vi "Exp1.vi"() -> ()   [LabVIEW 2016]
panel:
  out "R Value":dbl
  in  "3rd Band":string
  in  "2nd Band":string
  in  "1st Band":string
  out "Y":dbl
  in  "X":dbl
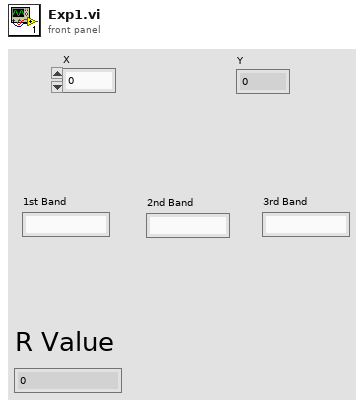
[diagram p1: front panel]
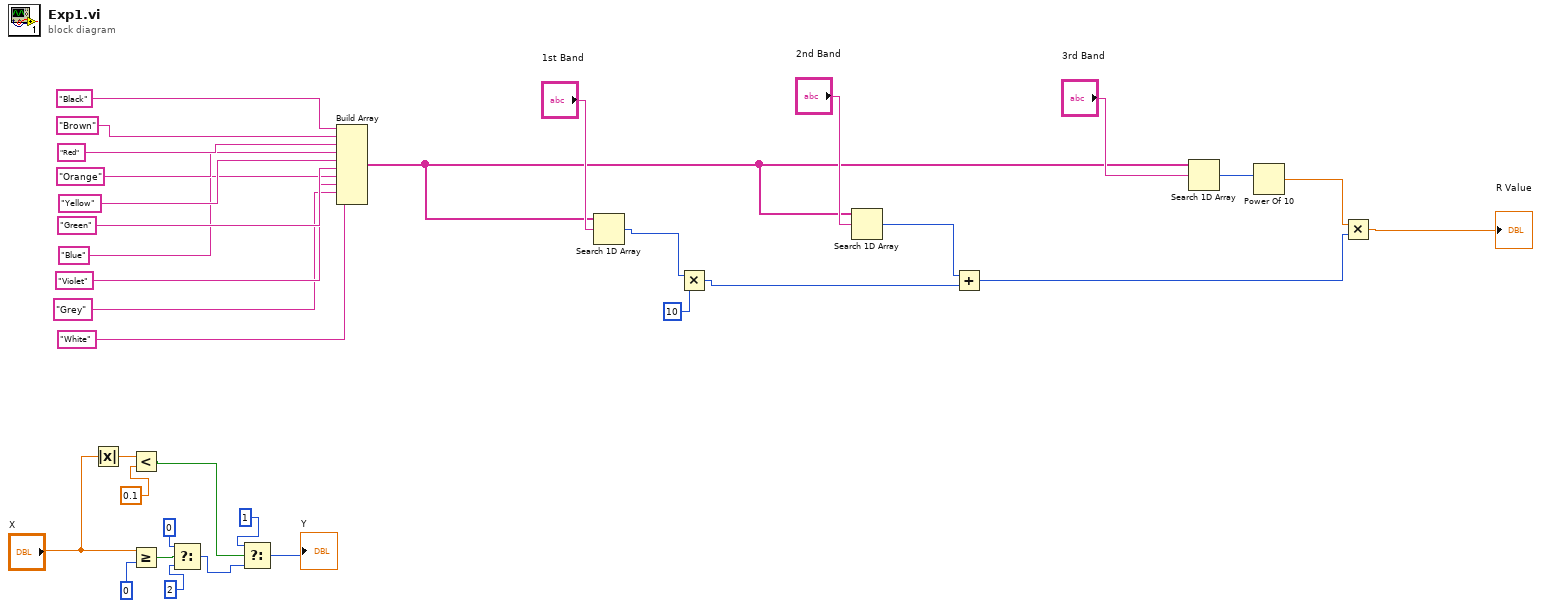
[diagram p0: block diagram]
diagram:
  n1 = Absolute Value(x="X") -> (abs(x)=w25:dbl)
  n2 = Less?(x=w25, y=0.1) -> (x < y?=w23:bool)
  n3 = Greater Or Equal?(x="X", y=0) -> (x >= y?=w27:bool)
  n4 = Select(t=0, s=w27, f=2) -> (s? t:f=w32:i32)
  n5 = Select(t=1, s=w23, f=w32) -> (s? t:f=→"Y":i32)
  n6 = Build Array("Black", "Brown", "Red", "Orange", "Yellow", "Green", "Blue", "Violet", "Grey", "White") -> (w6:string[])
  n7 = Search 1D Array(1D array=w6, element="1st Band") -> (index of element=w5:i32)  [unwired: 1 in]
  n8 = Multiply(x=w5, y=10) -> (x*y=w2:i32)
  n9 = Search 1D Array(1D array=w6, element="2nd Band") -> (index of element=w3:i32)  [unwired: 1 in]
  n10 = Add(x=w3, y=w2) -> (x+y=w1:i32)
  n11 = Search 1D Array(1D array=w6, element="3rd Band") -> (index of element=w12:i32)  [unwired: 1 in]
  n12 = Power Of 10(x=w12) -> (10^x=w11:dbl)
  n13 = Multiply(x=w11, y=w1) -> (x*y=→"R Value":dbl)
